vi "PRNG.vi"(8 "z":dbl[](array[numeric]), 9 "y":dbl[](array[numeric]), 10 "x":dbl[](array[numeric]), 11 "Numeric":i32) -> (0 "z":dbl[](array[numeric]), 1 "y":dbl[](array[numeric]), 2 "x":dbl[](array[numeric]))   [LabVIEW 2019]
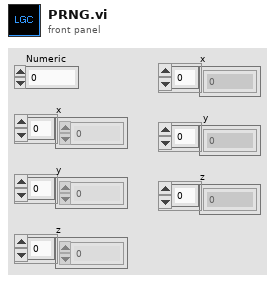
[diagram p1: front panel]
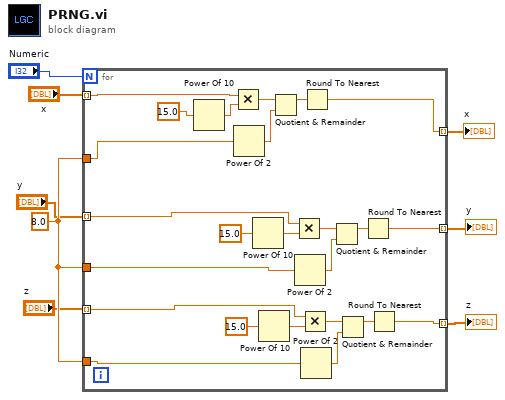
[diagram p0: block diagram]
diagram:
  w4 = 8.0
  n1 = for {
    N: "Numeric" -> [_]
    tunnel: w4 -> [w15]
    tunnel: [w9] -> w6 mode=indexing
    tunnel: w4 -> [w13]
    tunnel: w4 -> [w11]
    tunnel: [w18] -> w5 mode=indexing
    tunnel: [w16] -> w7 mode=indexing
    tunnel: "x" -> [w29] mode=indexing
    tunnel: "y" -> [w28] mode=indexing
    tunnel: "z" -> [w27] mode=indexing
    n2 = Power Of 10(x=15.0) -> (10^x=w25:dbl)
    n3 = Multiply(x=w29, y=w25) -> (x*y=w32:dbl)
    n4 = Power Of 2(x=w15) -> (2^x=w14:dbl)
    n5 = Power Of 10(x=15.0) -> (10^x=w23:dbl)
    n6 = Power Of 10(x=15.0) -> (10^x=w21:dbl)
    n7 = Quotient & Remainder(x=w32, y=w14) -> (x-y*floor(x/y)=w20:dbl)  [unwired: 1 out]
    n8 = Multiply(x=w28, y=w23) -> (x*y=w31:dbl)
    n9 = Power Of 2(x=w13) -> (2^x=w12:dbl)
    n10 = Multiply(x=w27, y=w21) -> (x*y=w30:dbl)
    n11 = Power Of 2(x=w11) -> (2^x=w10:dbl)
    n12 = Round To Nearest(number=w20) -> (nearest integer value=w9:dbl)
    n13 = Quotient & Remainder(x=w31, y=w12) -> (x-y*floor(x/y)=w19:dbl)  [unwired: 1 out]
    n14 = Quotient & Remainder(x=w30, y=w10) -> (x-y*floor(x/y)=w17:dbl)  [unwired: 1 out]
    n15 = Round To Nearest(number=w19) -> (nearest integer value=w18:dbl)
    n16 = Round To Nearest(number=w17) -> (nearest integer value=w16:dbl)
  }
  "z" <- w7
  "x" <- w6
  "y" <- w5
